vi "StringArray Create (String Length).vi"(8 "error in (no error)":errorcluster, 9 "String length":i32, 10 "Number of strings":i32, 11 "String array in":string) -> (0 "error out":errorcluster, 3 "StringArray DVR out":refnum<data-value>)   [LabVIEW 2012, in "MDSplus.lvlib"]
uses:
  <vilib>/MDSplus/Library/MDSplus.lvlib
  <vilib>/MDSplus/Classes/Data_Class/Array_Class/StringArray_Class/StringArray.lvclass
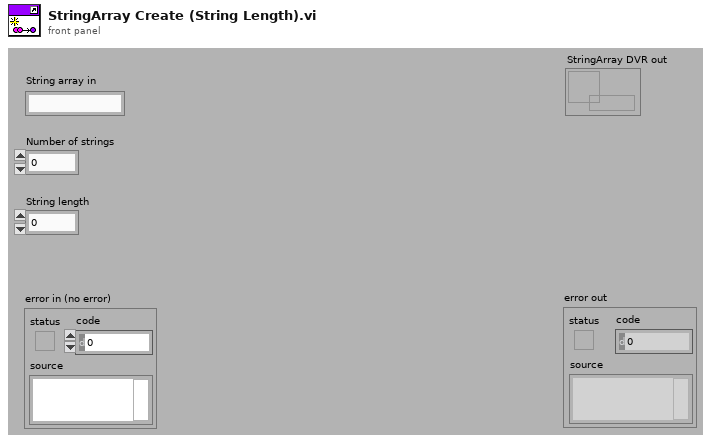
[diagram p1: front panel]
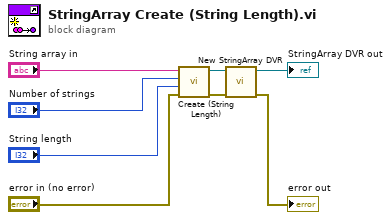
[diagram p0: block diagram]
diagram:
  n1 = call <vilib>:"Create (String Length).vi"("error in (no error)"="error in (no error)", "String length"="String length", "Number of strings"="Number of strings", "String array in"="String array in") -> ("error out"=w6:errorcluster, "StringArray out"=w7:refnum<class "StringArray.lvclass">)  [unwired: 6 in]
  n2 = call <vilib>:"New StringArray DVR.vi"("error in (no error)"=w6, "StringArray in"=w7) -> ("error out"=→"error out":errorcluster, "StringArray DVR out"=→"StringArray DVR out":refnum<data-value>)  [unwired: 8 in]
